vi "SE5082_Initialize.vi"(8 "error in (no error)":errorcluster, 9 "Reset (True)":bool, 10 "ID Query (True)":bool=TRUE, 11 "VISA resource name":refnum<visa-resource-name>) -> (0 "error out":errorcluster, 3 "VISA resource name out":refnum<visa-resource-name>)   [LabVIEW 2017]
doc: "Establishes communication with the instrument and optionally performs an instrument identification query and/or an instrument reset. It also places the instrument in a default state needed for other instrument driver operations. Therefore, call this VI before calling other instrument driver VIs for this instrument. Generally, you need to call the Initialize VI only once at the beginning of an application."
panel:
  out "IDN":string
  out "Instrument Information":T1
  # "(c) 2011-2013 National Instruments.  ALL RIGHTS RESERVED."
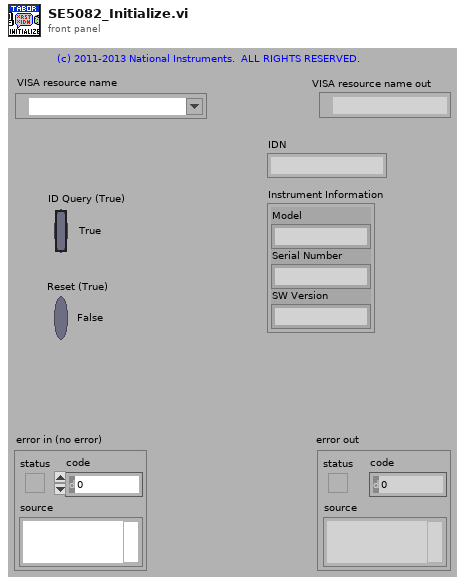
[diagram p1: front panel]
types:
  T1 = cluster{"Model":string, "Serial Number":string, "SW Version":string}
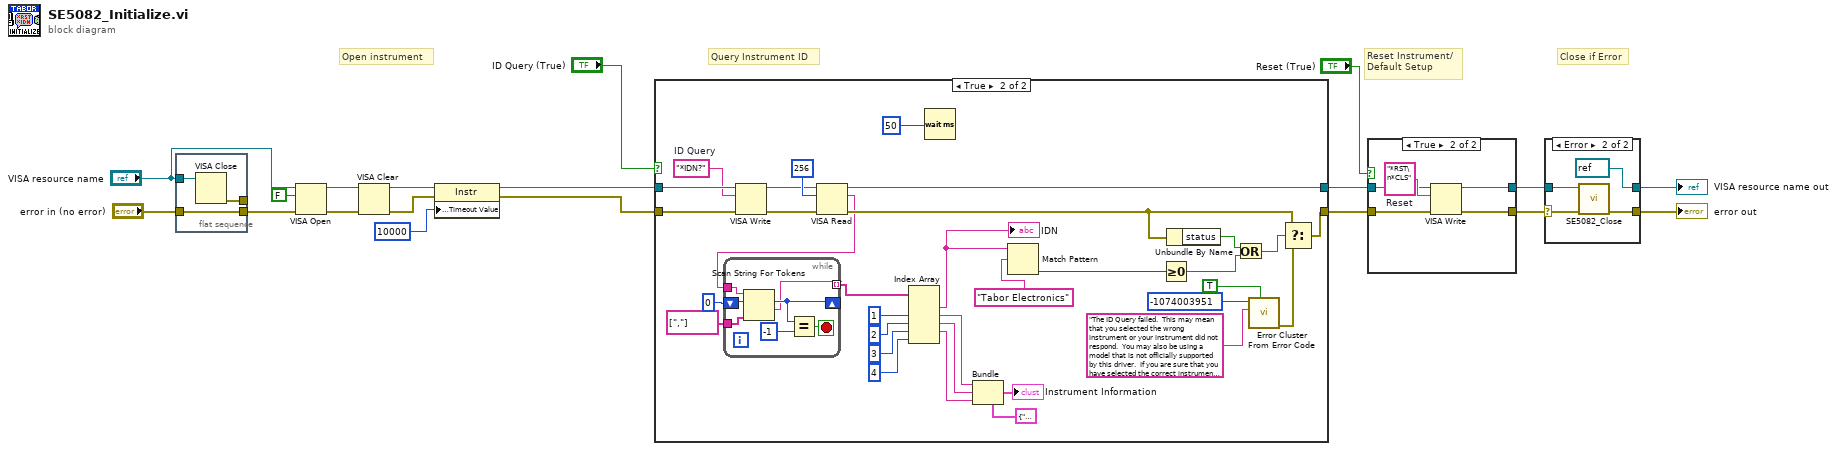
[diagram p0: block diagram]
diagram:
  # "Close if Error"
  # "Query Instrument ID"
  # "Reset Instrument/\nDefault Setup"
  # "Open instrument"
  n1 = flat-sequence {
    tunnel: "VISA resource name" -> [w22]
    tunnel: "error in (no error)" -> [w21]
    tunnel: [w21] -> w3
    tunnel: [w20] -> _
    frame #0 {
      n2 = VISA Close(VISA resource name=w22) -> (error out=w20:errorcluster)  [unwired: 1 in]
    }
  }
  n3 = VISA Open(duplicate session (F)=FALSE, error in (no error)=w3, VISA resource name="VISA resource name") -> (VISA resource name=w14:refnum<visa-resource-name>, error out=w13:errorcluster)  [unwired: 1 in, 1 out]
  n4 = VISA Clear(VISA resource name=w14, error in (no error)=w13) -> (VISA resource name out=w12:refnum<visa-resource-name>, error out=w11:errorcluster)
  n5 = property class="Instr"(reference=w12, error in=w11, "General Settings:Timeout Value"=u32 10000) -> (reference out=w6:refnum<visa-resource-name>, error out=w5:errorcluster)
  n6 = case shown="True" "ID Query (True)" {
    tunnel: [w23 w57] -> w18
    tunnel: [w24 w56] -> w19
    tunnel: w6 -> [w24 w53]
    tunnel: w5 -> [w23 w51]
    frame False {
    }
    frame True {
      w49 = "*IDN?"  # ID Query
      n7 = VISA Write(VISA resource name=w53, write buffer=w49, error in (no error)=w51) -> (VISA resource name out=w52:refnum<visa-resource-name>, error out=w50:errorcluster)  [unwired: 1 out]
      n8 = VISA Read(VISA resource name=w52, byte count=u32 256, error in (no error)=w50) -> (VISA resource name out=w56:refnum<visa-resource-name>, read buffer=w35:string, error out=w54:errorcluster)  [unwired: 1 out]
      n9 = while {
        shift-right: [w62] -> _
        shift-left: 0 ("offset past token") -> [w64]
        tunnel: [w60] -> w38 mode=indexing
        tunnel: w35 -> [w59]
        tunnel: string[] [","] ("delimiters (\\s,\\t,\\r,\\n)") -> [w58]
        stop <- w63 stop-if-true
        n10 = Scan String For Tokens(6:w58, 8:w64, 9:w59) -> (1:w60:string, 2:w62:i32)  [unwired: 3 in, 2 out]
        n11 = Equal?(x=w62, y=-1) -> (x = y?=w63:bool)
      }
      n12 = Index Array(array=w38, index #2=1 ("index"), index #3=2 ("index"), index #4=3 ("index"), index #5=4 ("index")) -> (element #1=w25:string, element #2=w44:string, element #3=w45:string, element #4=w46:string)  [unwired: 1 in, 1 out]
      "IDN" <- w25
      n13 = Wait (ms)(milliseconds to wait=u32 50 ("Delay (500ms)")) -> ()  [unwired: 1 out]
      n14 = Bundle(cluster=T1 {"Model"="", "Serial Number"="", "SW Version"=""} ("Instrument Information"), "Model"=w44, "Serial Number"=w45, "SW Version"=w46) -> (→"Instrument Information":T1)
      n15 = Match Pattern(string=w25, regular expression="Tabor Electronics") -> (offset past match=w26:i32)  [unwired: 1 in, 3 out]
      n16 = Greater Or Equal To 0?(x=w26) -> (x >= 0?=w29:bool)
      n17 = Unbundle By Name(w54) -> ("status"=w30:bool)
      n18 = Or(x=w30, y=w29) -> (x .or. y?=w28:bool)
      n19 = call <vilib>:"Error Cluster From Error Code.vi"("show call chain? (False)"=TRUE, "error message (\"\")"="The ID Query failed.  This may mean that you selected the wrong instrument or your instrument did not respond.  You may also be using a model that is not officially supported by this driver.  If you are sure that you have selected the correct instrument and it is responding, try disabling the ID Query." ("Source (VI Name)"), "error code (0)"=-1074003951 ("Code")) -> ("error out"=w34:errorcluster)  [unwired: 1 in, 5 out]
      n20 = Select(t=w54, s=w28, f=w34) -> (s? t:f=w57:errorcluster)
    }
  }
  n21 = case shown="True" "Reset (True)" {
    tunnel: w18 -> [w66 w70]
    tunnel: [w66 w69] -> w7
    tunnel: w19 -> [w65 w67]
    tunnel: [w65 w68] -> w8
    frame False {
    }
    frame True {
      w71 = "*RST\n*CLS"  # Reset
      n22 = VISA Write(VISA resource name=w67, write buffer=w71, error in (no error)=w70) -> (VISA resource name out=w68:refnum<visa-resource-name>, error out=w69:errorcluster)  [unwired: 1 out]
    }
  }
  n23 = case shown="Error" w7 {
    selector: w7 -> [w72 w75]
    tunnel: w8 -> [w73 w76]
    tunnel: [w73 refnum<visa-resource-name> refnum ("VISA resource name out")] -> w10
    tunnel: [w72 w77] -> w9
    frame No Error {
    }
    frame Error {
      n24 = call "SE5082_Close.vi"("error in (no error)"=w75, "VISA resource name"=w76) -> ("error out"=w77:errorcluster)  [unwired: 9 in]
    }
  }
  "VISA resource name out" <- w10
  "error out" <- w9
